vi "runtest filter instruments to be used.vi"(4 "ixStep":i32, 5 "Step Number":i32, 6 "sxStationId":string, 7 "POST (empty)":T2, 8 "error in (no error)":errorcluster, 9 "Instruments In":T3[](array[typedef]), 10 "Instrument Types":string[](array[string]), 11 "Connection Refnum":T1) -> (0 "error out":errorcluster, 2 "Instruments Out":T3[](array[typedef]), 3 "Connection Refnum":T1)   [LabVIEW 2011]
uses:
  server/database/Stations/Instruments/Instrument Record.ctl
  Addons/internet/utils/keyedarr.llb/Keyed Array.ctl
  SI.LIB/ODBC/SQL Controls/Connection Refnum.ctl
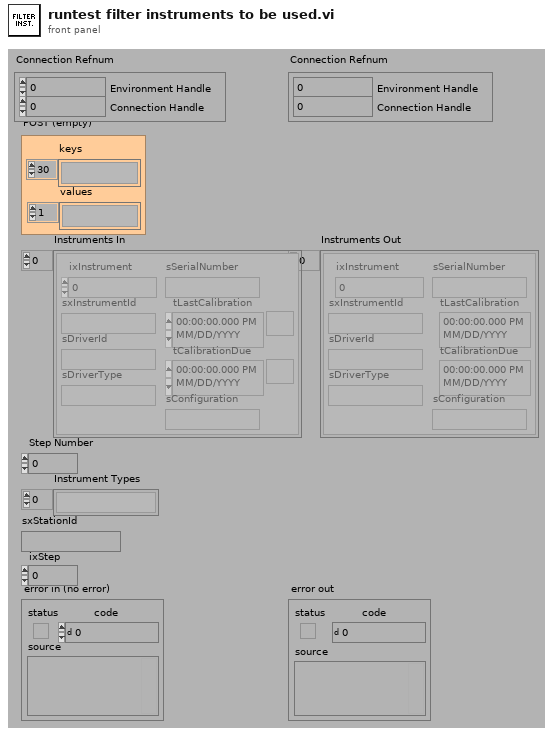
[diagram p1: front panel]
types:
  T1 = typedef "Connection Refnum.ctl" = cluster{"Environment Handle":i32, "Connection Handle":i32}
  T2 = typedef "Keyed Array.ctl" = cluster{"keys":string[], "values":string[]}
  T3 = typedef "Instrument Record.ctl" = cluster{"ixInstrument":i32, "sxInstrumentId":string, "sDriverId":string, "sDriverType":string, "sSerialNumber":string, "tLastCalibration":timestamp, "tCalibrationDue":timestamp, "sConfiguration":string}
  T4 = typedef "Station Record.ctl" = cluster{"ixStation":i32, "sxStationId":string, "sIP":string, "fVerified":bool}
  T5 = typedef "Step Association Record.ctl" = cluster{"ixStepAssociation":i32, "iStep":i32, "iStation":i32, "iInstrument":i32}
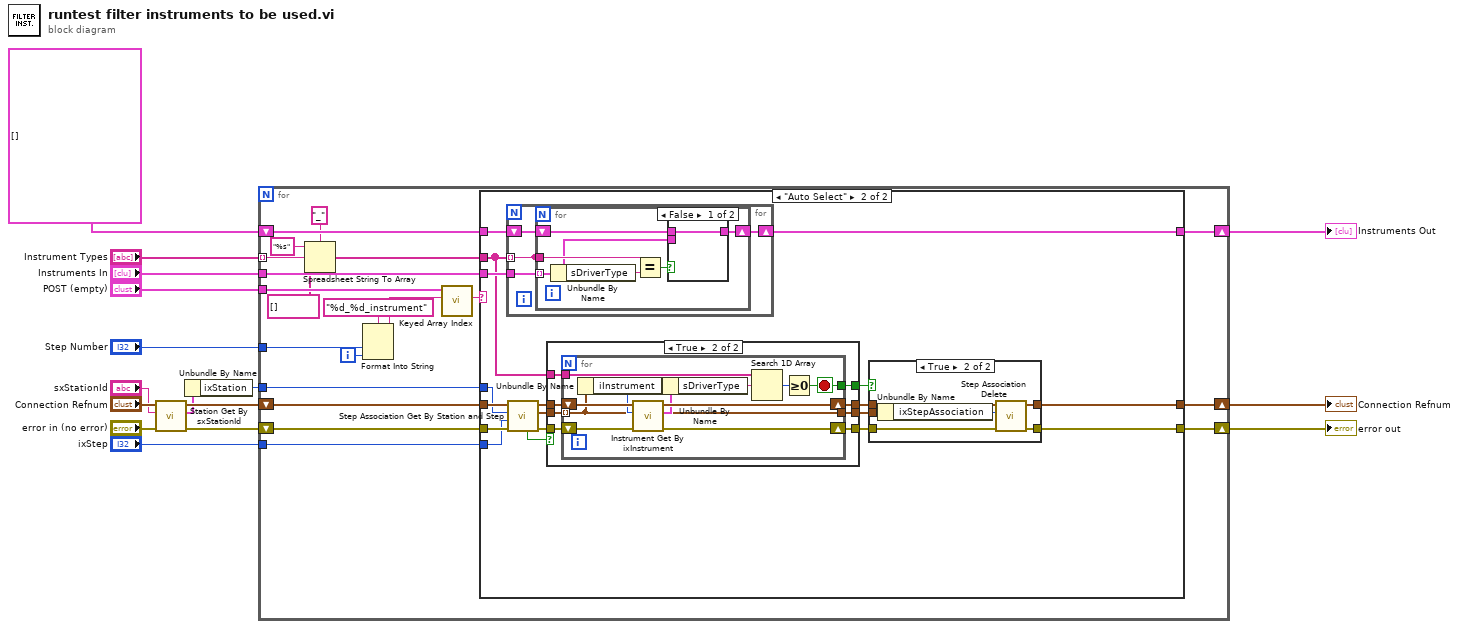
[diagram p0: block diagram]
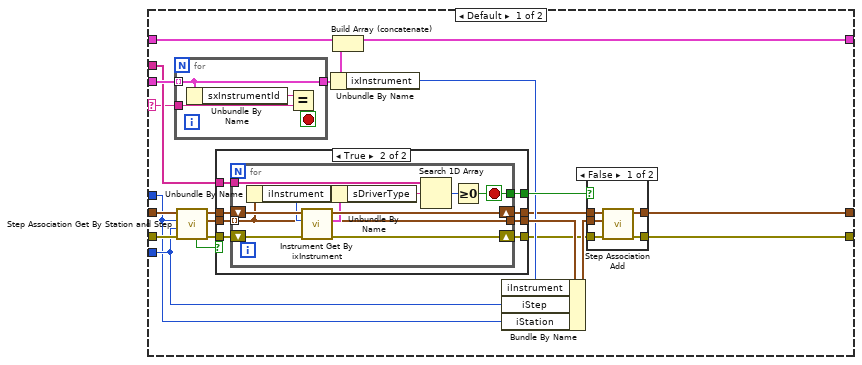
[diagram p2: hidden frame]
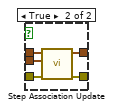
[diagram p3: hidden frame]
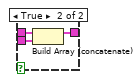
[diagram p7: hidden frame]
diagram:
  n1 = call "Station Get By sxStationId.vi"("error in (no error)"="error in (no error)", "sxStationId (\"\")"="sxStationId", "Connection Refnum"="Connection Refnum") -> ("error out"=w6:errorcluster, "Station Record"=w3:T4, "Connection Refnum"=w7:T1)  [unwired: 4 in, 2 out]
  n2 = Unbundle By Name(w3) -> ("ixStation"=w1:i32)
  n3 = for {
    tunnel: "POST (empty)" -> [w35]
    tunnel: "Step Number" -> [w36]
    tunnel: "Instruments In" -> [w34]
    shift-right: [w32] -> w12
    shift-left: T3[] [] ("Instruments In") -> [w33]
    tunnel: "Instrument Types" -> [w18] mode=indexing
    shift-right: [w27] -> w4
    shift-left: w7 -> [w31]
    shift-right: [w26] -> w5
    shift-left: w6 -> [w30]
    tunnel: "ixStep" -> [w29]
    tunnel: w1 -> [w28]
    i -> [w22]
    n4 = Spreadsheet String To Array(delimiter (Tab)="_", format string="%s", spreadsheet string=w18, array type (2D Dbl)=string[] []) -> (array=w17:string[])
    n5 = Format Into String(format string="%d_%d_instrument", w36, w22) -> (resulting string=w24:string)  [unwired: 2 in, 1 out]
    n6 = call "Keyed Array Index.vi"("key"=w24, "array in"=w35) -> ("value"=w23:string)  [unwired: 2 in, 3 out]
    n7 = case shown="\"Auto Select\"" w23 {
      selector: w23 -> [w47 _]
      tunnel: w34 -> [w58 w111]
      tunnel: w33 -> [w57 w110]
      tunnel: [w56 w109] -> w32
      tunnel: w31 -> [w54 w100]
      tunnel: w30 -> [w55 w101]
      tunnel: w29 -> [w46 w97]
      tunnel: w28 -> [w45 w96]
      tunnel: [w42 w99] -> w27
      tunnel: [w41 w98] -> w26
      tunnel: w17 -> [w50 w95]
      frame Default {
        n8 = for {
          tunnel: w58 -> [w90] mode=indexing
          tunnel: w47 -> [w93]
          tunnel: [w90] -> w37
          stop <- w91 stop-if-true
          n9 = Unbundle By Name(w90) -> ("sxInstrumentId"=w92:string)
          n10 = Equal?(x=w92, y=w93) -> (x = y?=w91:bool)
        }
        n11 = call "Step Association Get By Station and Step.vi"("error in (no error)"=w55, "iStep (0)"=w46, "iStation (0)"=w45, "Connection Refnum"=w54) -> ("error out"=w52:errorcluster, "Step Associations"=w49:T5[], "Connection Refnum"=w53:T1, "Data Present?"=w51:bool)  [unwired: 4 in]
        n12 = case shown="True" w51 {
          tunnel: w53 -> [w70 w77]
          tunnel: w52 -> [w69 w76]
          tunnel: [w70 w74] -> w38
          tunnel: [w69 w73] -> w39
          tunnel: w50 -> [_ w75]
          tunnel: w49 -> [_ w78]
          tunnel: [_ w72] -> w48
          tunnel: [_ w71] -> w44
          frame False {
          }
          frame True {
            n13 = for {
              tunnel: w78 -> [w80] mode=indexing
              shift-right: [w88] -> w73
              shift-left: w76 -> [w89]
              shift-right: [w87] -> w74
              shift-left: w77 -> [w86]
              tunnel: w75 -> [w83]
              tunnel: [w80] -> w71
              tunnel: [w79] -> w72
              stop <- w79 stop-if-true
              n14 = Unbundle By Name(w80) -> ("iInstrument"=w85:i32)
              n15 = call "Instrument Get By ixInstrument.vi"("error in (no error)"=w89, "ixInstrument"=w85, "Connection Refnum"=w86) -> ("error out"=w88:errorcluster, "Instrument Record"=w84:T3, "Connection Refnum"=w87:T1)  [unwired: 5 in, 1 out]
              n16 = Unbundle By Name(w84) -> ("sDriverType"=w82:string)
              n17 = Search 1D Array(1D array=w83, element=w82) -> (index of element=w81:i32)  [unwired: 1 in]
              n18 = Greater Or Equal To 0?(x=w81) -> (x >= 0?=w79:bool)
            }
          }
        }
        n19 = Unbundle By Name(w37) -> ("ixInstrument"=w40:i32)
        n20 = Build Array (concatenate)(w57, w37) -> (w56:T3[])
        n21 = Bundle By Name(cluster=w44, "iInstrument"=w40, "iStep"=w46, "iStation"=w45) -> (w43:T5)
        n22 = case shown="False" w48 {
          tunnel: w43 -> [w63 w68]
          tunnel: w39 -> [w59 w67]
          tunnel: w38 -> [w60 w66]
          tunnel: [w61 w65] -> w42
          tunnel: [w62 w64] -> w41
          frame False {
            n23 = call "Step Association Add.vi"("error in (no error)"=w59, "Step Association Record (empty)"=w63, "Connection Refnum"=w60) -> ("error out"=w62:errorcluster, "Connection Refnum"=w61:T1)  [unwired: 7 in]
          }
          frame True {
            n24 = call "Step Association Update.vi"("error in (no error)"=w67, "Step Association Record (empty)"=w68, "Connection Refnum"=w66) -> ("error out"=w64:errorcluster, "Connection Refnum"=w65:T1)  [unwired: 7 in]
          }
        }
      }
      frame "Auto Select" {
        n25 = for {
          tunnel: w95 -> [w141] mode=indexing
          tunnel: w111 -> [w144]
          shift-right: [w142] -> w109
          shift-left: w110 -> [w143]
          tunnel: [w141] -> _ mode=indexing
          n26 = for {
            tunnel: w144 -> [w145] mode=indexing
            tunnel: w141 -> [w150]
            shift-right: [w146] -> w142
            shift-left: w143 -> [w147]
            n27 = Unbundle By Name(w145) -> ("sDriverType"=w149:string)
            n28 = Equal?(x=w150, y=w149) -> (x = y?=w148:bool)
            n29 = case shown="False" w148 {
              tunnel: [w151 w154] -> w146
              tunnel: w145 -> [_ w153]
              tunnel: w147 -> [w151 w152]
              frame False {
              }
              frame True {
                n30 = Build Array (concatenate)(w152, w153) -> (w154:T3[])
              }
            }
          }
        }
        n31 = call "Step Association Get By Station and Step.vi"("error in (no error)"=w101, "iStep (0)"=w97, "iStation (0)"=w96, "Connection Refnum"=w100) -> ("error out"=w107:errorcluster, "Step Associations"=w105:T5[], "Connection Refnum"=w108:T1, "Data Present?"=w106:bool)  [unwired: 4 in]
        n32 = case shown="True" w106 {
          tunnel: w108 -> [w121 w128]
          tunnel: w107 -> [w120 w127]
          tunnel: [w121 w125] -> w102
          tunnel: [w120 w124] -> w103
          tunnel: w95 -> [_ w126]
          tunnel: w105 -> [_ w129]
          tunnel: [_ w123] -> w104
          tunnel: [_ w122] -> w94
          frame False {
          }
          frame True {
            n33 = for {
              tunnel: w129 -> [w131] mode=indexing
              shift-right: [w139] -> w124
              shift-left: w127 -> [w140]
              shift-right: [w138] -> w125
              shift-left: w128 -> [w137]
              tunnel: w126 -> [w134]
              tunnel: [w131] -> w122
              tunnel: [w130] -> w123
              stop <- w130 stop-if-true
              n34 = Unbundle By Name(w131) -> ("iInstrument"=w136:i32)
              n35 = call "Instrument Get By ixInstrument.vi"("error in (no error)"=w140, "ixInstrument"=w136, "Connection Refnum"=w137) -> ("error out"=w139:errorcluster, "Instrument Record"=w135:T3, "Connection Refnum"=w138:T1)  [unwired: 5 in, 1 out]
              n36 = Unbundle By Name(w135) -> ("sDriverType"=w133:string)
              n37 = Search 1D Array(1D array=w134, element=w133) -> (index of element=w132:i32)  [unwired: 1 in]
              n38 = Greater Or Equal To 0?(x=w132) -> (x >= 0?=w130:bool)
            }
          }
        }
        n39 = case shown="True" w104 {
          tunnel: w94 -> [_ w115]
          tunnel: w103 -> [w112 w119]
          tunnel: w102 -> [w113 w118]
          tunnel: [w113 w117] -> w99
          tunnel: [w112 w116] -> w98
          frame False {
          }
          frame True {
            n40 = Unbundle By Name(w115) -> ("ixStepAssociation"=w114:i32)
            n41 = call "Step Association Delete.vi"("error in (no error)"=w119, "ixStepAssociation (0)"=w114, "Connection Refnum"=w118) -> ("error out"=w116:errorcluster, "Connection Refnum"=w117:T1)  [unwired: 7 in]
          }
        }
      }
    }
  }
  "Instruments Out" <- w12
  "error out" <- w5
  "Connection Refnum" <- w4
